vi "load_hyst_data.vi"() -> (0 "Hyst(U_nom)":dbl[](array[numeric]), 1 "U_nom":dbl[](array[numeric]), 2 "wp":dbl[](array[numeric]), 3 "rps":dbl[](array[numeric]), 4 "N_sat":i32)   [LabVIEW 2017, in "Sat_Hyst_TestCase.lvclass"]
uses:
  Sat_Hyst_TestCase.lvclass
  <vilib>/Utility/file.llb/Read Delimited Spreadsheet (DBL).vi
panel:
  out "all rows":dbl[][](array[numeric])
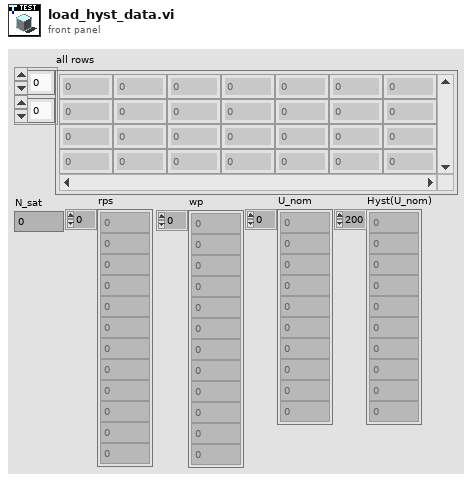
[diagram p1: front panel]
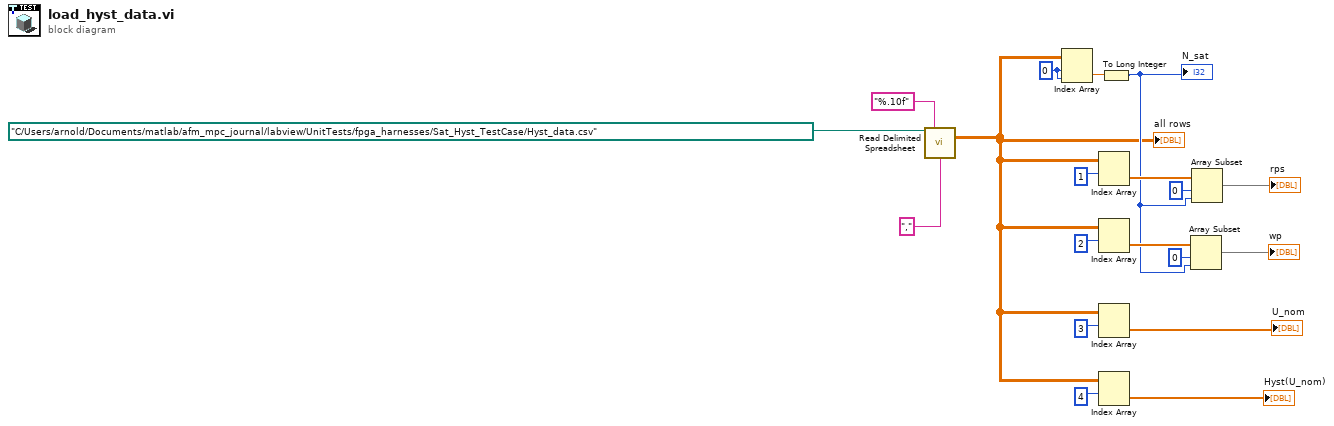
[diagram p0: block diagram]
diagram:
  w17 = 0 ("index (row)")
  n1 = call-poly <vilib>:"Read Delimited Spreadsheet.vi"("file path (dialog if empty)"=path "C:/Users/arnold/Documents/matlab/afm_mpc_journal/labview/UnitTests/fpga_harnesses/Sat_Hyst_TestCase/Hyst_data.csv" ("Path"), "format (%.3f)"="%.10f", "delimiter (\\t)"="," ("delimiter (\\t)")) -> ("all rows"=w4:dbl[][])  [unwired: 7 in, 5 out]
  "all rows" <- w4
  n2 = Index Array(array=w4, index (row)=w17, index (col)=w17) -> (element=w10:dbl)
  n3 = Index Array(array=w4, index (row)=1) -> (element=w15:dbl[])  [unwired: 1 in]
  n4 = Index Array(array=w4, index (row)=2) -> (element=w12:dbl[])  [unwired: 1 in]
  n5 = Index Array(array=w4, index (row)=3) -> (element=→"U_nom":dbl[])  [unwired: 1 in]
  n6 = Index Array(array=w4, index (row)=4) -> (element=→"Hyst(U_nom)":dbl[])  [unwired: 1 in]
  n7 = To Long Integer(number=w10) -> (32bit integer=w9:i32)
  "N_sat" <- w9
  n8 = Array Subset(array=w12, index=0, length=w9) -> (→"wp":dbl[])
  n9 = Array Subset(array=w15, index=0, length=w9) -> (→"rps":dbl[])
